vi "Close Ref.vi"(8 "error in (no error)":errorcluster, 11 "Agilent 33210A in":refnum<class "Agilent 33210A.lvclass">) -> (0 "error out":errorcluster, 3 "Agilent 33210A out":refnum<class "Agilent 33210A.lvclass">)   [LabVIEW 2021, in "Func Generator.lvlib" / "Agilent 33210A.lvclass"]
uses:
  Agilent 33210A.lvclass
  Agilent 33210A.lvclass/Agilent 33210A.ctl
  <instrlib>/Agilent 33XXX Series/Agilent 33XXX Series.lvlib
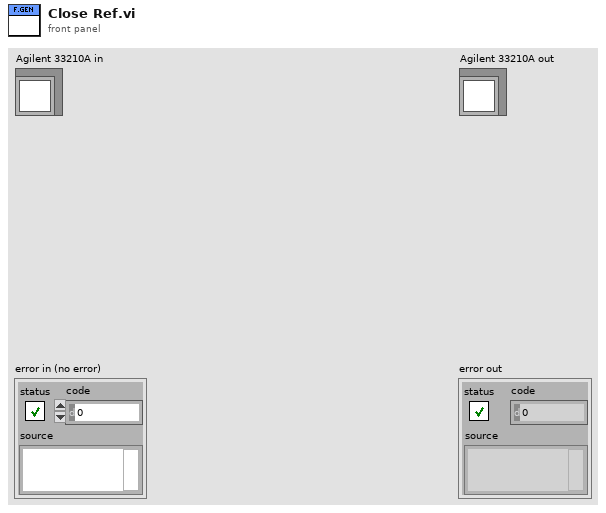
[diagram p1: front panel]
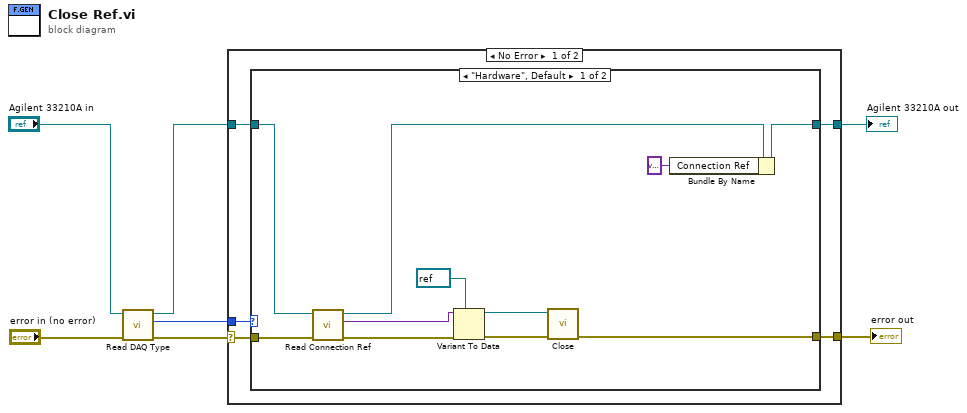
[diagram p0: block diagram]
diagram:
  n1 = call-dynamic "Read DAQ Type.vi"("error in (no error)"="error in (no error)", "Agilent 33210A in"="Agilent 33210A in") -> ("error out"=w6:errorcluster, "DAQ Type"=w5:enum16{"Hardware", "Simulation"}, "Agilent 33210A out"=w1:refnum<class "Agilent 33210A.lvclass">)  [unwired: 7 in]
  n2 = case shown="No Error" w6 {
    selector: w6 -> [w12 w26]
    tunnel: w5 -> [w11 _]
    tunnel: w1 -> [w10 w27]
    tunnel: [w9 w27] -> w3
    tunnel: [w8 w26] -> w2
    frame No Error {
      n3 = case shown="\"Hardware\", Default" w11 {
        tunnel: w12 -> [w23 w24]
        tunnel: w10 -> [w14 w25]
        tunnel: [w16 w25] -> w9
        tunnel: [w17 w24] -> w8
        frame "Hardware", Default {
          n4 = call-dynamic "Read Connection Ref.vi"("error in (no error)"=w23, "Agilent 33210A in"=w14) -> ("error out"=w22:errorcluster, "Connection Ref"=w21:variant, "Agilent 33210A out"=w13:refnum<class "Agilent 33210A.lvclass">)  [unwired: 7 in]
          n5 = Variant To Data(error in=w22, type=refnum<visa-resource-name> refnum ("VISA resource name"), Variant=w21) -> (data=w19:refnum<visa-resource-name>, error out=w18:errorcluster)
          n6 = call <instrlib>:"Close.vi"("error in (no error)"=w18, "VISA resource name"=w19) -> ("error out"=w17:errorcluster)  [unwired: 9 in]
          n7 = Bundle By Name(cluster=w13, "Connection Ref"=variant) -> (w16:refnum<class "Agilent 33210A.lvclass">)
        }
        frame "Simulation" {
        }
      }
    }
    frame Error {
    }
  }
  "error out" <- w2
  "Agilent 33210A out" <- w3
